vi "DAQmx Create Channel (CI-Position-Linear Encoder).vi"(0 "task in":refnum<k21>, 1 "z index enable":bool, 2 "z index value":dbl, 3 "z index phase":i32(ring)=10040 items=["A High B High"=10040, "A High B Low"=10041, "A Low B High"=10042, "A Low B Low"=10043], 5 "counter":tag, 6 "decoding type":i32(ring)=10092 items=["X1"=10090, "X2"=10091, "X4"=10092, "Two Pulse Counting"=10313], 7 "name to assign":string, 9 "units":i32(ring)=10219 items=["Meters"=10219, "Inches"=10379, "Ticks"=10304, "From Custom Scale"=10065], 11 "error in":errorcluster, 12 "custom scale name":tag, 13 "distance per pulse":dbl=0.001, 14 "initial position":dbl) -> (4 "task out":refnum<k21>, 15 "error out":errorcluster)   [LabVIEW 2013]
doc: "Creates a channel that uses a linear encoder to measure linear position. With the exception of devices that support multi-counter tasks, you can create only one counter input channel at a time with this VI because a task can contain only one counter input channel. To read from multiple counters simultaneously, use a separate task for each counter. Connect the input signals to the default input terminals of the counter unless you select different input terminals."
uses:
  <resource>/objmgr/daqmx.rc
panel:
  # "z index info"
  # "encoder info"
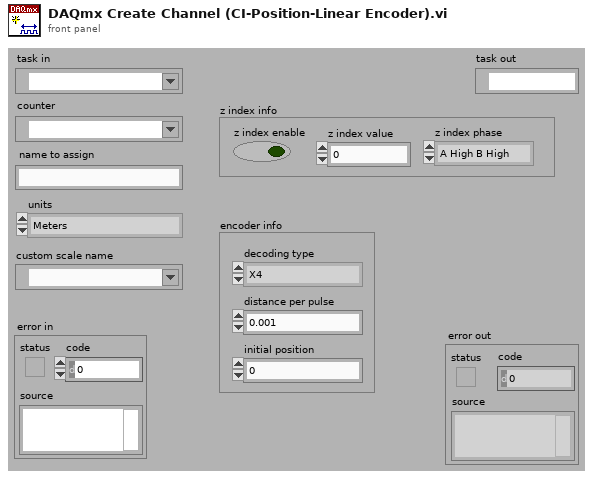
[diagram p1: front panel]
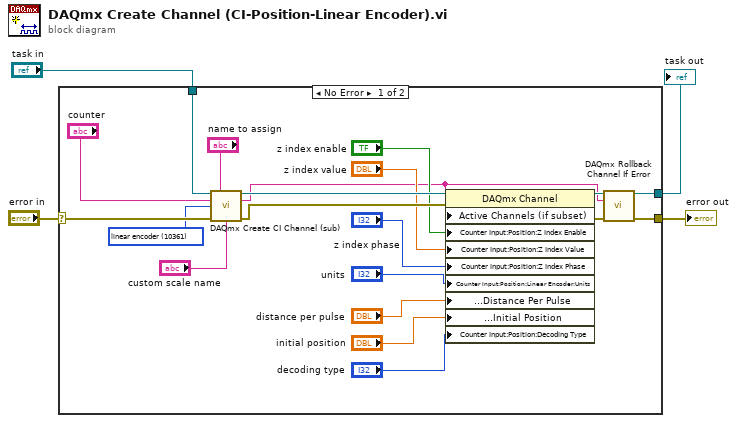
[diagram p0: block diagram]
diagram:
  n1 = case shown="No Error" "error in" {
    selector: "error in" -> [w23 w25]
    tunnel: "task in" -> [w24 w26]
    tunnel: [w17 w26] -> w2
    tunnel: [w16 w25] -> w1
    frame No Error {
      w14 = 10361 items=["count events"=10125, "frequency"=10179, "period"=10256, "pulse width"=10359, "semi period"=10289, "two edge separation"=10267, "angular encoder"=10360, "linear encoder"=10361] ("measurement type")
      n2 = call "DAQmx Create CI Channel (sub).vi"("task in"=w24, "virtual channel name"="name to assign", "physical channel name"="counter", "measurement type"=w14, "error in"=w23, "custom scale"="custom scale name") -> ("task out"=w19:refnum<k21>, "channel names"=w6:string, "error out"=w21:errorcluster)  [unwired: 7 out]
      n3 = property class="DAQmx Channel"(reference=w19, error in=w21, "Active Channels (if subset)"=w6, "Counter Input:Position:Z Index Enable"="z index enable", "Counter Input:Position:Z Index Value"="z index value", "Counter Input:Position:Z Index Phase"="z index phase", "Counter Input:Position:Linear Encoder:Units"="units", "Counter Input:Position:Linear Encoder:Distance Per Pulse"="distance per pulse", "Counter Input:Position:Linear Encoder:Initial Position"="initial position", "Counter Input:Position:Decoding Type"="decoding type") -> (reference out=w18:refnum<k21>, error out=w15:errorcluster)
      n4 = call "DAQmx Rollback Channel If Error.vi"("task in"=w18, "channel names"=w6, "error in"=w15) -> ("task out"=w17:refnum<k21>, "error out"=w16:errorcluster)  [unwired: 11 out]
    }
    frame Error {
    }
  }
  "error out" <- w1
  "task out" <- w2
